vi "String to Number.vi"(9 "length":i32, 10 "offset":i32, 11 "string":string) -> (3 "numeric":dbl)   [LabVIEW 2017, in "GW Instek PSP-405.lvlib"]
doc: "Converts <b>string</b> command response into a double precision float."
uses:
  GW Instek PSP-405.lvlib
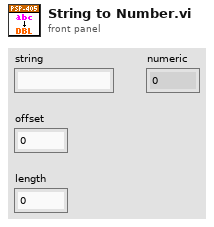
[diagram p1: front panel]
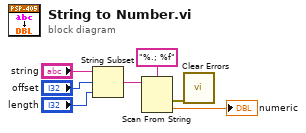
[diagram p0: block diagram]
diagram:
  n1 = String Subset(string="string", offset (0)="offset", length (rest)="length") -> (substring=w4:string)
  n2 = Scan From String(format string="%.; %f", input string=w4) -> (error out=w1:errorcluster, output 1=→"numeric":dbl)  [unwired: 3 in, 2 out]
  n3 = call <vilib>:"Clear Errors.vi"("error in (no error)"=w1) -> ()  [unwired: 5 in, 2 out]
